vi "VRM_GoToField_SubVI.vi"(8 "error in (no error)":errorcluster, 10 "Wait until reach setpoint?":bool=TRUE, 11 "VRM Targets":T1={"X Setpoint (T)"=0.0, "Y Setpoint (T)"=0.0, "Z Setpoint (T)"=0.0, "Sweep Rate (T/min)"=0.1}) -> (0 "error out":errorcluster)   [LabVIEW 2016]
doc: "USE AT YOUR OWN RISK!\nThis subVI is meant to be called as a subVI of \"Mercury_GoToField.vi\", which will take care of the persistent switch for you"
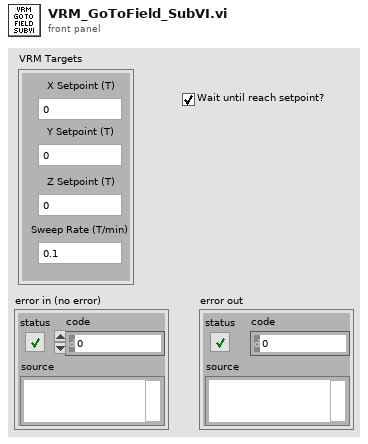
[diagram p1: front panel]
types:
  T1 = cluster{"X Setpoint (T)":dbl, "Y Setpoint (T)":dbl, "Z Setpoint (T)":dbl, "Sweep Rate (T/min)":dbl}
  T2 = cluster{"Hold":bool, "Clamp":bool, "To Set":bool, "To Zero":bool, "Send to IPS":bool}
  T3 = cluster{"X Target (T)":dbl, "Y Target (T)":dbl, "Z Target (T)":dbl, "X Field (T)":dbl, "Y Field (T)":dbl, "Z Field (T)":dbl, "X Rate (T/min)":dbl, "Y Rate (T/min)":dbl, "Z Rate (T/min)":dbl, "X Current (A)":dbl, "Y Current (A)":dbl, "Z Current (A)":dbl, "X Voltage (V)":dbl, "Y Voltage (V)":dbl, "Z Voltage (V)":dbl}
  T4 = cluster{"x action":string, "y action":string, "z action":string}
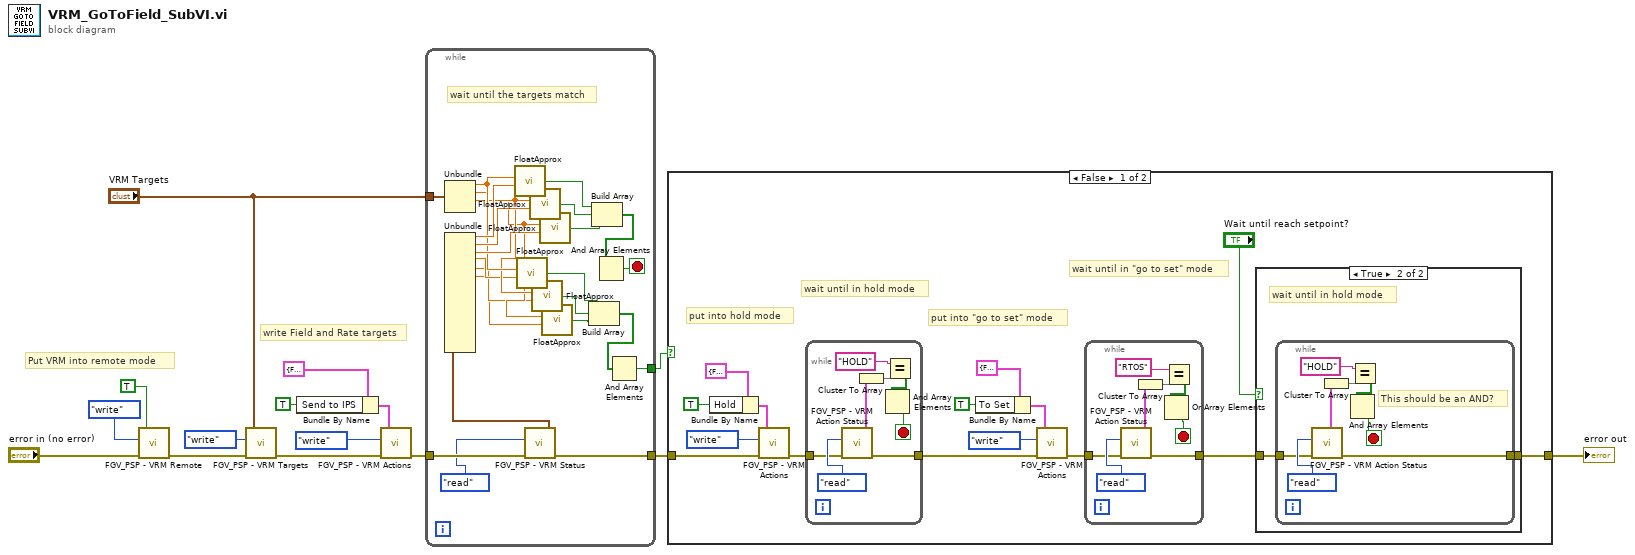
[diagram p0: block diagram]
diagram:
  # "Put VRM into remote mode"
  # "write Field and Rate targets"
  n1 = call "FGV_PSP - VRM Remote.vi"("error in"="error in (no error)", "Function"=enum16{"write", "read"}."write", "VRM Remote"=TRUE ("Mercury Remote")) -> ("error out"=w6:errorcluster)  [unwired: 3 in, 1 out]
  n2 = call "FGV_PSP - VRM Targets.vi"("error in"=w6, "Function"=enum16{"write", "read"}."write", "VRM Targets"="VRM Targets") -> ("error out"=w12:errorcluster)  [unwired: 3 in, 1 out]
  n3 = Bundle By Name(cluster=T2 {"Hold"=FALSE, "Clamp"=FALSE, "To Set"=FALSE, "To Zero"=FALSE, "Send to IPS"=FALSE} ("VRM actions"), "Send to IPS"=TRUE) -> (w3:T2)
  n4 = call "FGV_PSP - VRM Actions.vi"("error in"=w12, "Function"=enum16{"write", "read"}."write", "VRM actions"=w3) -> ("error out"=w13:errorcluster)  [unwired: 3 in, 1 out]
  n5 = while {
    tunnel: w13 -> [w39]
    tunnel: "VRM Targets" -> [w38]
    tunnel: [w37] -> w14
    tunnel: [w34] -> w1
    stop <- w33 stop-if-true
    # "wait until the targets match"
    n6 = Unbundle(w38) -> ("X Setpoint (T)"=w25:dbl, "Y Setpoint (T)"=w24:dbl, "Z Setpoint (T)"=w23:dbl)  [unwired: 1 out]
    n7 = call "FGV_PSP - VRM Status.vi"("error in"=w39, "Function"=enum16{"write", "read"}."read") -> ("error out"=w37:errorcluster, "VRM status"=w35:T3)  [unwired: 4 in]
    n8 = Unbundle(w35) -> ("X Target (T)"=w32:dbl, "Y Target (T)"=w31:dbl, "Z Target (T)"=w30:dbl, "X Field (T)"=w22:dbl, "Y Field (T)"=w21:dbl, "Z Field (T)"=w20:dbl)  [unwired: 9 out]
    n9 = call "FloatApprox.vi"("y"=w32, "x"=w25) -> ("x ~ y?"=w27:bool)  [unwired: 2 in]
    n10 = call "FloatApprox.vi"("y"=w22, "x"=w25) -> ("x ~ y?"=w17:bool)  [unwired: 2 in]
    n11 = call "FloatApprox.vi"("y"=w31, "x"=w24) -> ("x ~ y?"=w28:bool)  [unwired: 2 in]
    n12 = call "FloatApprox.vi"("y"=w21, "x"=w24) -> ("x ~ y?"=w18:bool)  [unwired: 2 in]
    n13 = call "FloatApprox.vi"("y"=w30, "x"=w23) -> ("x ~ y?"=w29:bool)  [unwired: 2 in]
    n14 = call "FloatApprox.vi"("y"=w20, "x"=w23) -> ("x ~ y?"=w19:bool)  [unwired: 2 in]
    n15 = Build Array(w17, w18, w19) -> (w16:bool[])
    n16 = Build Array(w27, w28, w29) -> (w26:bool[])
    n17 = And Array Elements(Boolean array=w26) -> (logical AND=w33:bool)
    n18 = And Array Elements(Boolean array=w16) -> (logical AND=w34:bool)
  }
  n19 = case shown="False" w1 {
    tunnel: [w53 w82] -> w15
    tunnel: w14 -> [w51 w82]
    frame False {
      # "wait until in \"go to set\" mode"
      # "put into \"go to set\" mode"
      # "wait until in hold mode"
      # "put into hold mode"
      n20 = Bundle By Name(cluster=T2 {"Hold"=FALSE, "Clamp"=FALSE, "To Set"=FALSE, "To Zero"=FALSE, "Send to IPS"=FALSE} ("VRM actions"), "Hold"=TRUE ("Send to IPS")) -> (w46:T2)
      n21 = call "FGV_PSP - VRM Actions.vi"("error in"=w51, "Function"=enum16{"write", "read"}."write", "VRM actions"=w46) -> ("error out"=w50:errorcluster)  [unwired: 3 in, 1 out]
      n22 = while {
        tunnel: w50 -> [w80]
        tunnel: [w79] -> w52
        stop <- w75 stop-if-true
        n23 = call "FGV_PSP - VRM Action Status.vi"("error in"=w80, "Function"=enum16{"write", "read"}."read") -> ("error out"=w79:errorcluster, "VRM Actions"=w74:T4)  [unwired: 4 in]
        n24 = Cluster To Array(cluster=w74) -> (array=w77:string[])
        n25 = Equal?(x="HOLD" ("x action"), y=w77) -> (x = y?=w76:bool[])
        n26 = And Array Elements(Boolean array=w76) -> (logical AND=w75:bool)
      }
      n27 = Bundle By Name(cluster=T2 {"Hold"=FALSE, "Clamp"=FALSE, "To Set"=FALSE, "To Zero"=FALSE, "Send to IPS"=FALSE} ("VRM actions"), "To Set"=TRUE ("Send to IPS")) -> (w45:T2)
      n28 = call "FGV_PSP - VRM Actions.vi"("error in"=w52, "Function"=enum16{"write", "read"}."write", "VRM actions"=w45) -> ("error out"=w49:errorcluster)  [unwired: 3 in, 1 out]
      n29 = while {
        tunnel: w49 -> [w72]
        tunnel: [w71] -> w54
        stop <- w67 stop-if-true
        n30 = call "FGV_PSP - VRM Action Status.vi"("error in"=w72, "Function"=enum16{"write", "read"}."read") -> ("error out"=w71:errorcluster, "VRM Actions"=w70:T4)  [unwired: 4 in]
        n31 = Cluster To Array(cluster=w70) -> (array=w69:string[])
        n32 = Equal?(x="RTOS" ("x action"), y=w69) -> (x = y?=w66:bool[])
        n33 = Or Array Elements(Boolean array=w66) -> (logical OR=w67:bool)
      }
      n34 = case shown="True" "Wait until reach setpoint?" {
        tunnel: w54 -> [w55 w57]
        tunnel: [w55 w56] -> w53
        frame False {
        }
        frame True {
          # "wait until in hold mode"
          n35 = while {
            tunnel: w57 -> [w64]
            tunnel: [w63] -> w56
            stop <- w58 stop-if-true
            # "This should be an AND?"
            n36 = call "FGV_PSP - VRM Action Status.vi"("error in"=w64, "Function"=enum16{"write", "read"}."read") -> ("error out"=w63:errorcluster, "VRM Actions"=w59:T4)  [unwired: 4 in]
            n37 = Cluster To Array(cluster=w59) -> (array=w61:string[])
            n38 = Equal?(x="HOLD" ("x action"), y=w61) -> (x = y?=w62:bool[])
            n39 = And Array Elements(Boolean array=w62) -> (logical AND=w58:bool)
          }
        }
      }
    }
    frame True {
      # "Don't do you anything if you are already at setpoint"
    }
  }
  "error out" <- w15
